vi "segmentation test.vi"() -> ()   [LabVIEW 2009]
panel:
  in  "divisor increment":i32=1
  out "Waveform Graph":dbl[](graph)
  in  "iterations":i32(slide) scale=0.0..1000.0
  in  "time (s)":dbl
  in  "acceleration (m/s/s)":dbl(slide) scale=0.0..10.0
  # "displays the final distance as the segmentation of time increases.  (It's a function of the accuracy of the floating poit datatype as the divisor is increased and re-multiplied."
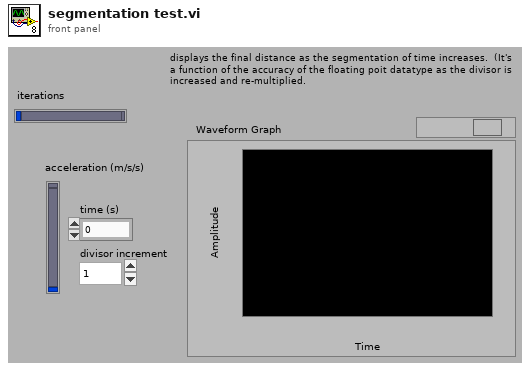
[diagram p1: front panel]
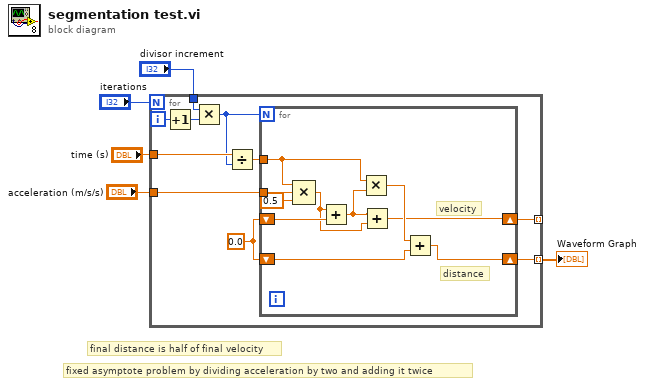
[diagram p0: block diagram]
diagram:
  # "fixed asymptote problem by dividing acceleration by two and adding it twice"
  # "final distance is half of final velocity"
  n1 = for {
    N: "iterations" -> [_]
    tunnel: "time (s)" -> [w14]
    tunnel: "acceleration (m/s/s)" -> [w13]
    tunnel: [w11] -> w1 mode=indexing
    tunnel: [w9] -> _ mode=indexing
    tunnel: "divisor increment" -> [w6]
    i -> [w15]
    w10 = 0.0
    n2 = Increment(x=w15) -> (x+1=w8:i32)
    n3 = Multiply(x=w6, y=w8) -> (x*y=w7:i32)
    n4 = Divide(x=w14, y=w7) -> (x/y=w12:dbl)
    n5 = for {
      N: w7 -> [_]
      tunnel: w13 -> [w25]
      tunnel: w12 -> [w23]
      shift-right: [w16] -> w9
      shift-left: w10 -> [w24]
      shift-right: [w20] -> w11
      shift-left: w10 -> [w21]
      # "distance"
      # "velocity"
      n6 = Compound Arithmetic op=MULTIPLY(w23, w25, 0.5 ("value")) -> (w17:dbl)
      n7 = Add(x=w17, y=w24) -> (x+y=w18:dbl)
      n8 = Multiply(x=w23, y=w18) -> (x*y=w22:dbl)
      n9 = Add(x=w18, y=w17) -> (x+y=w16:dbl)
      n10 = Add(x=w22, y=w21) -> (x+y=w20:dbl)
    }
  }
  "Waveform Graph" <- w1
